vi "simpletest.vi"() -> ()   [LabVIEW 2020]
uses:
  <vilib>/VIPM Community/HTTP Client Plugin - NI Advanced/Classes/HTTP Client Advanced/HTTP Client Advanced.lvclass
  C:/Program Files/National Instruments/LabVIEW 2025/vi.lib/VIPM Community/HTTP Client Plugin - Base/Classes/Abstract HTTP Client/Abstract HTTP Client.lvclass
  <vilib>/VIPM Community/HTTP Client Plugin - Base/Classes/LabVIEW HTTP Client/LabVIEW HTTP Client.lvclass
  labview-rs-reqwest/lv_src/HTTP Client Plugin/HTTP Client reqwest.lvclass
  classes/REST Client/REST Client.lvclass
  classes/Response Headers/Response Headers.lvclass
panel:
  out "Array 2":dbl[][](array[numeric])
  out "Array":string[][](array[string])
  # "TOTAL\nhead\nget\npost\nput\npatch"
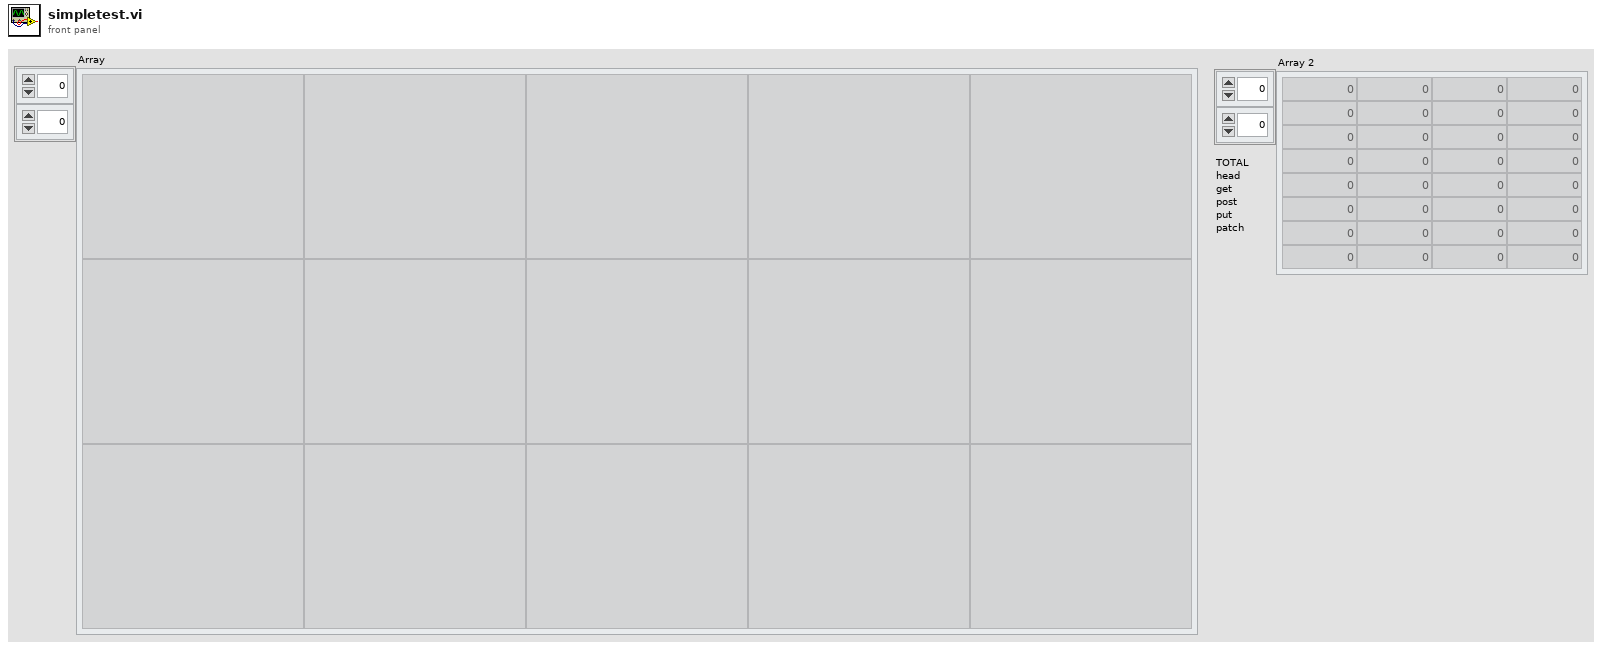
[diagram p1: front panel]
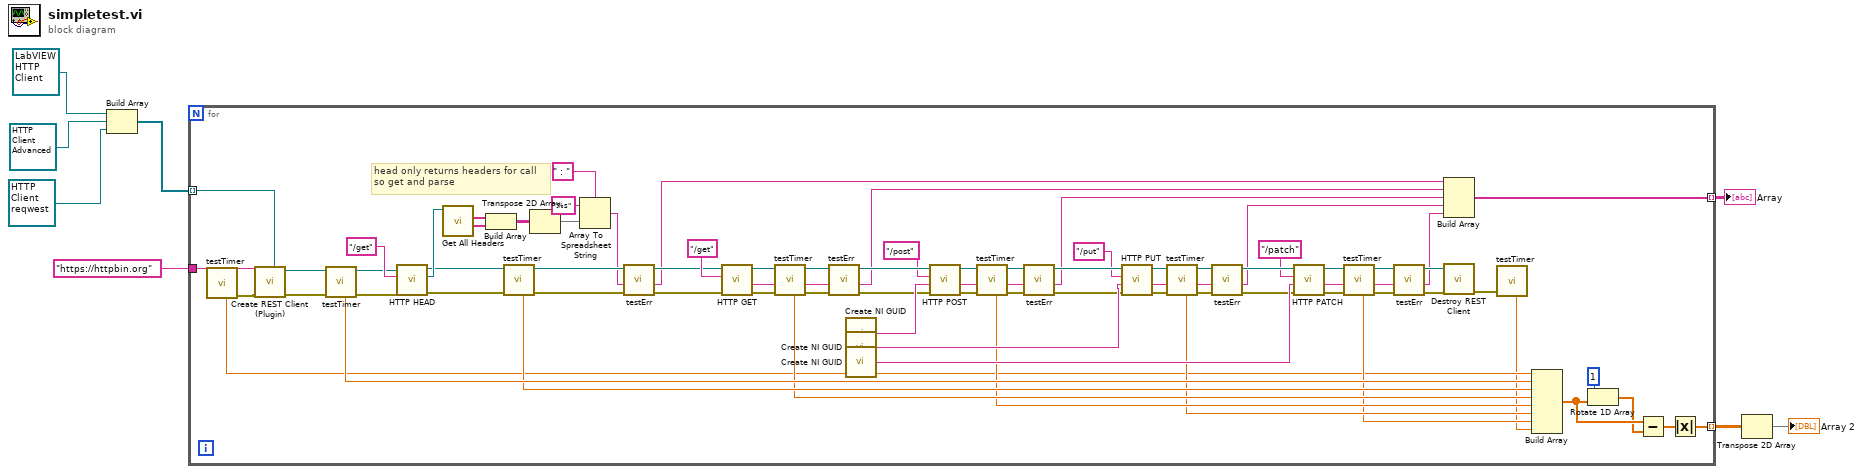
[diagram p0: block diagram]
diagram:
  n1 = Build Array(refnum<class "LabVIEW HTTP Client.lvclass"> refnum ("HTTP Client Abstract.lvlib:LabVIEW HTTP Client.lvclass"), refnum<class "HTTP Client Advanced.lvclass"> refnum ("HTTP Client Advanced in"), refnum<class "HTTP Client reqwest.lvclass"> refnum ("HTTP Client reqwest.lvclass")) -> (w2:refnum<class "Abstract HTTP Client.lvclass">[])
  n2 = for {
    tunnel: [w51] -> w8 mode=indexing
    tunnel: [w11] -> w7 mode=indexing
    tunnel: "https://httpbin.org" ("Base URL") -> [w10]
    tunnel: w2 -> [w9] mode=indexing
    # "head only returns headers for call\nso get and parse"
    n3 = call "testTimer.vi"() -> ("error out"=w19:errorcluster, "relative seconds"=w18:dbl)  [unwired: 10 in]
    n4 = call "Create REST Client (Plugin).vi"("http-client-type"=w9, "error in (no error)"=w19, "Base URL"=w10) -> ("error out"=w65:errorcluster, "REST Client out"=w66:refnum<class "REST Client.lvclass">)  [unwired: 7 in]
    n5 = call "testTimer.vi"("error in (no error)"=w65) -> ("error out"=w30:errorcluster, "relative seconds"=w25:dbl)  [unwired: 9 in]
    n6 = call-dynamic "HTTP HEAD.vi"("error in (no error)"=w30, "Path"="/get", "REST Client in"=w66) -> ("error out"=w32:errorcluster, "Response Headers"=w72:refnum<class "Response Headers.lvclass">, "REST Client out"=w64:refnum<class "REST Client.lvclass">)  [unwired: 3 in, 3 out]
    n7 = call "Get All Headers.vi"("Response Headers in"=w72) -> ("Values"=w70:string[], "Names"=w71:string[])  [unwired: 7 in, 2 out]
    n8 = Build Array(w71, w70) -> (w69:string[][])
    n9 = call "testTimer.vi"("error in (no error)"=w32) -> ("error out"=w31:errorcluster, "relative seconds"=w24:dbl)  [unwired: 9 in]
    n10 = Transpose 2D Array(2D array=w69) -> (transposed array=w68:string[][])
    n11 = Array To Spreadsheet String(delimiter (Tab)=" : ", array=w68, 3:"%s" ("format string")) -> (spreadsheet string=w46:string)
    n12 = call "testErr.vi"("error in (no error)"=w31, "OutputString"=w46) -> ("error out"=w47:errorcluster, "TestStr"=w45:string)  [unwired: 8 in]
    n13 = call-dynamic "HTTP GET.vi"("error in (no error)"=w47, "Path"="/get", "REST Client in"=w64) -> ("error out"=w61:errorcluster, "Response body"=w43:string, "REST Client out"=w62:refnum<class "REST Client.lvclass">)  [unwired: 3 in, 3 out]
    n14 = call "testTimer.vi"("error in (no error)"=w61) -> ("error out"=w29:errorcluster, "relative seconds"=w23:dbl)  [unwired: 9 in]
    n15 = call "testErr.vi"("error in (no error)"=w29, "OutputString"=w43) -> ("error out"=w44:errorcluster, "TestStr"=w42:string)  [unwired: 8 in]
    n16 = call <vilib>:"Create NI GUID.vi"() -> ("NI GUID"=w50:string)
    n17 = call <vilib>:"Create NI GUID.vi"() -> ("NI GUID"=w49:string)
    n18 = call <vilib>:"Create NI GUID.vi"() -> ("NI GUID"=w48:string)
    n19 = call-dynamic "HTTP POST.vi"("error in (no error)"=w44, "Request body"=w50, "Path"="/post", "REST Client in"=w62) -> ("error out"=w59:errorcluster, "Response body"=w40:string, "REST Client out"=w60:refnum<class "REST Client.lvclass">)  [unwired: 2 in, 3 out]
    n20 = call "testTimer.vi"("error in (no error)"=w59) -> ("error out"=w28:errorcluster, "relative seconds"=w22:dbl)  [unwired: 9 in]
    n21 = call "testErr.vi"("error in (no error)"=w28, "OutputString"=w40) -> ("error out"=w41:errorcluster, "TestStr"=w39:string)  [unwired: 8 in]
    n22 = call-dynamic "HTTP PUT.vi"("error in (no error)"=w41, "Request body"=w49, "Path"="/put", "REST Client in"=w60) -> ("error out"=w57:errorcluster, "Response body"=w37:string, "REST Client out"=w58:refnum<class "REST Client.lvclass">)  [unwired: 2 in, 3 out]
    n23 = call "testTimer.vi"("error in (no error)"=w57) -> ("error out"=w27:errorcluster, "relative seconds"=w21:dbl)  [unwired: 9 in]
    n24 = call "testErr.vi"("error in (no error)"=w27, "OutputString"=w37) -> ("error out"=w38:errorcluster, "TestStr"=w36:string)  [unwired: 8 in]
    n25 = call-dynamic "HTTP PATCH.vi"("error in (no error)"=w38, "Request body"=w48, "Path"="/patch", "REST Client in"=w58) -> ("error out"=w55:errorcluster, "Response body"=w34:string, "REST Client out"=w56:refnum<class "REST Client.lvclass">)  [unwired: 2 in, 3 out]
    n26 = call "testTimer.vi"("error in (no error)"=w55) -> ("error out"=w26:errorcluster, "relative seconds"=w20:dbl)  [unwired: 9 in]
    n27 = call "testErr.vi"("error in (no error)"=w26, "OutputString"=w34) -> ("error out"=w35:errorcluster, "TestStr"=w33:string)  [unwired: 8 in]
    n28 = Build Array(w45, w42, w39, w36, w33) -> (w51:string[])
    n29 = call-dynamic "Destroy REST Client.vi"("error in (no error)"=w35, "REST Client in"=w56) -> ("error out"=w17:errorcluster)  [unwired: 9 in]
    n30 = call "testTimer.vi"("error in (no error)"=w17) -> ("relative seconds"=w16:dbl)  [unwired: 9 in, 1 out]
    n31 = Build Array(w18, w25, w24, w23, w22, w21, w20, w16) -> (w15:dbl[])
    n32 = Rotate 1D Array(1:w15, 2:1 ("n")) -> (0:w14:dbl[])
    n33 = Subtract(x=w15, y=w14) -> (x-y=w13:dbl[])
    n34 = Absolute Value(x=w13) -> (abs(x)=w11:dbl[])
  }
  "Array" <- w8
  n35 = Transpose 2D Array(2D array=w7) -> (transposed array=→"Array 2":dbl[][])
